vi "Read File.vi"(8 "error in (no error)":errorcluster, 11 "Context in":T1 {"Progress" scale=0.0..100.0}) -> (0 "error out":errorcluster, 3 "Context out":T1 {"Progress" scale=0.0..100.0})   [LabVIEW 2020, in "DocTool.lvlib"]
uses:
  DocTool.lvlib
  TDefs/Context.ctl
  Events.ctl
  UserEvent.ctl
  TDefs/State.ctl
  TDefs/States.ctl
  TDefs/Single File Properties.ctl
  TDefs/FP Items Properties.ctl
  TDefs/FP Item Properties.ctl
  TDefs/CopyTag.ctl
  StateMachine.lvlib
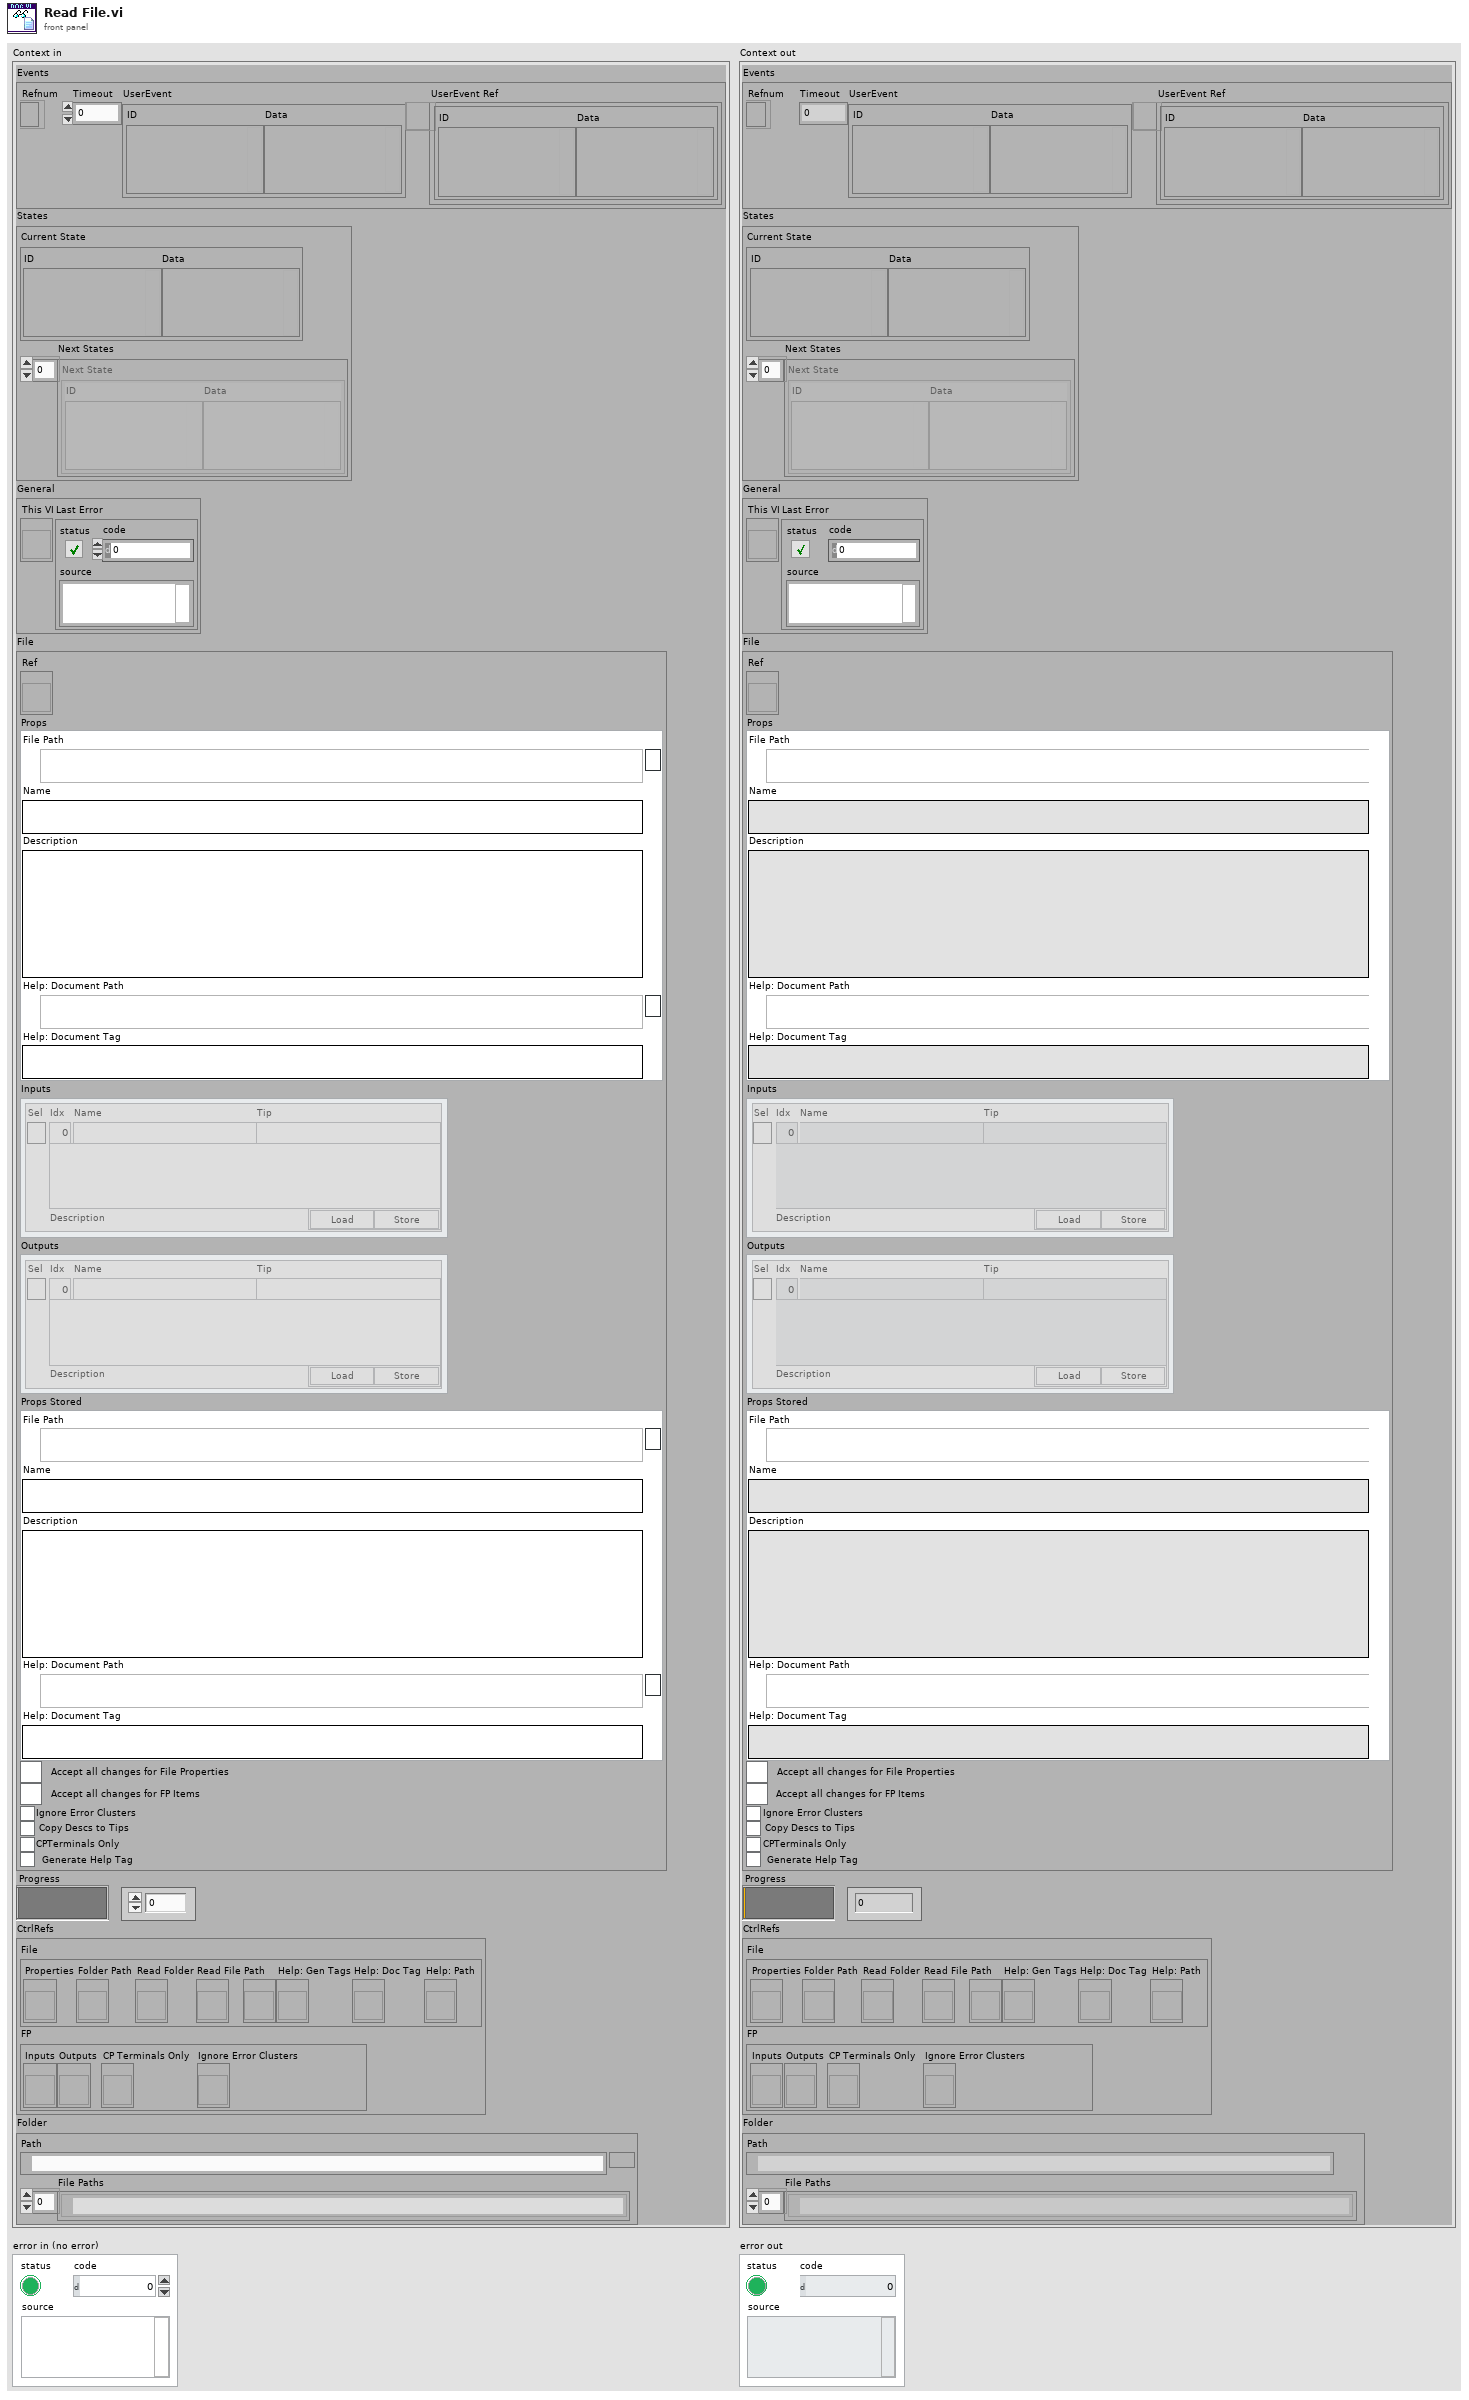
[diagram p1: front panel]
types:
  T1 = typedef "DocTool.lvlib/Context.ctl" = cluster{"Events":T2, "States":cluster{"Current State":T4, "Next States":T5}, "General":cluster{"This VI":refnum<vi>, "Last Error":errorcluster}, "File":cluster{"Ref":refnum<vi>, "Props":T6, "Inputs":T7, "Outputs":T7, "Props Stored":T6, "Write":bool, "Write FP":bool, "Ignore Error Clusters":bool, "Copy Descs to Tips":bool, "CPTerminals Only":bool, "Generate Help Tag":bool}, "Progress":i32, "CtrlRefs":cluster{"File":cluster{"Properties":refnum<vi>, "Folder Path":refnum<vi>, "Read Folder":refnum<vi>, "Read File":refnum<vi>, "Path":refnum<vi>, "Help: Gen Tags":refnum<vi>, "Help: Doc Tag":refnum<vi>, "Help: Path":refnum<vi>}, "FP":cluster{"Inputs":refnum<vi>, "Outputs":refnum<vi>, "CP Terminals Only":refnum<vi>, "Ignore Error Clusters":refnum<vi>}}, "Folder":cluster{"Path":path, "File Paths":path[]}}
  T2 = typedef "StateMachine.lvlib/Events.ctl" = cluster{"Refnum":refnum<event-registration>, "Timeout":i32, "UserEvent":T3, "UserEvent Ref":refnum<user-event>}
  T3 = typedef "StateMachine.lvlib/UserEvent.ctl" = cluster{"ID":variant, "Data":variant}
  T4 = typedef "StateMachine.lvlib/State.ctl" = cluster{"ID":variant, "Data":variant}
  T5 = typedef "StateMachine.lvlib/States.ctl" = T4[]
  T6 = typedef "DocTool.lvlib/Single File Properties.ctl" = cluster{"File Path":path, "Name":string, "Description":string, "Help: Document Path":path, "Help: Document Tag":string}
  T7 = typedef "DocTool.lvlib/FP Items Properties.ctl" = T8[]
  T8 = typedef "DocTool.lvlib/FP Item Properties.ctl" = cluster{"Sel":bool, "Idx":i32, "Name":string, "Description":string, "Tip":string, "Load Store":T9}
  T9 = typedef "DocTool.lvlib/CopyTag.ctl" = cluster{"Load":bool, "Store":bool}
  T10 = enum8{"Enabled", "Disabled", "Disabled and Grayed Out"}
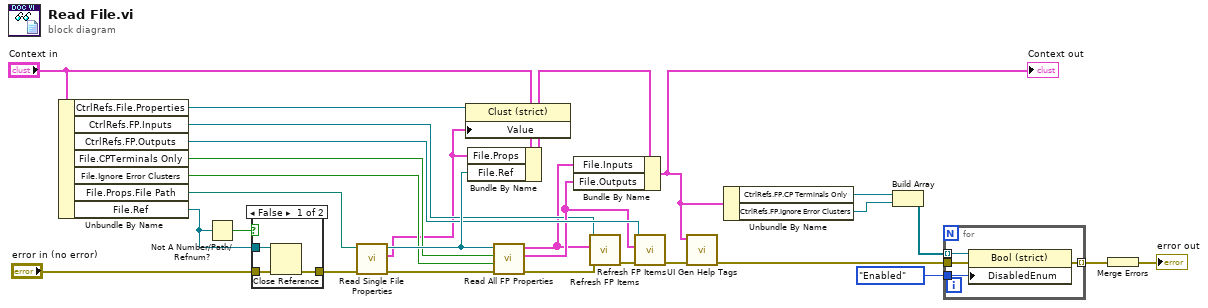
[diagram p0: block diagram]
diagram:
  n1 = Unbundle By Name("Context in") -> ("CtrlRefs.File.Properties"=w17:refnum<vi>, "CtrlRefs.FP.Inputs"=w20:refnum<vi>, "CtrlRefs.FP.Outputs"=w23:refnum<vi>, "File.CPTerminals Only"=w24:bool, "File.Ignore Error Clusters"=w26:bool, "File.Props.File Path"=w13:path, "File.Ref"=w10:refnum<vi>)
  n2 = Not A Number/Path/Refnum?(number/path/refnum=w10) -> (NaN/Path/Refnum?=w9:bool)
  n3 = case shown="False" w9 {
    tunnel: w10 -> [w31 _]
    tunnel: "error in (no error)" -> [w30 w32]
    tunnel: [w29 w32] -> w11
    frame False {
      n4 = Close Reference(reference=w31, error in (no error)=w30) -> (error out=w29:errorcluster)
    }
    frame True {
    }
  }
  n5 = call "Read Single File Properties.vi"("error in (no error)"=w11, "File Path"=w13) -> ("error out"=w15:errorcluster, "File Properties"=w18:T6, "File Ref"=w27:refnum<vi>)  [unwired: 7 in]
  n6 = property class="Clust (strict)"(reference=w17, "Value"=w18) -> ()  [unwired: 1 in, 2 out]
  n7 = Bundle By Name(cluster="Context in", "File.Props"=w18, "File.Ref"=w27) -> (w16:T1)
  n8 = call "Read All FP Properties.vi"("error in (no error)"=w15, "No Error clusters"=w26, "Is On Connector Pane"=w24, "VI in"=w27) -> ("error out"=w25:errorcluster, "Outputs"=w22:T7, "Inputs"=w19:T7)  [unwired: 5 in]
  n9 = Bundle By Name(cluster=w16, "File.Inputs"=w19, "File.Outputs"=w22) -> (w5:T1)
  "Context out" <- w5
  n10 = call "Refresh FP Items.vi"("error in (no error)"=w25, "FP Item Props in"=w19, "Array in"=w20) -> ("error out"=w21:errorcluster)  [unwired: 8 in]
  n11 = call "Refresh FP Items.vi"("error in (no error)"=w21, "FP Item Props in"=w22, "Array in"=w23) -> ("error out"=w28:errorcluster)  [unwired: 8 in]
  n12 = call "UI Gen Help Tags.vi"("error in (no error)"=w28, "Context"=w5) -> ("error out"=w4:errorcluster)  [unwired: 9 in]
  n13 = Unbundle By Name(w5) -> ("CtrlRefs.FP.CP Terminals Only"=w7:refnum<vi>, "CtrlRefs.FP.Ignore Error Clusters"=w3:refnum<vi>)
  n14 = Build Array(w7, w3) -> (w6:refnum<vi>[])
  n15 = for {
    tunnel: w6 -> [w36] mode=indexing
    tunnel: w4 -> [w35]
    tunnel: [w34] -> w2 mode=indexing
    tunnel: T10."Enabled" ("Disabled") -> [w33]
    n16 = property class="Bool (strict)"(reference=w36, error in=w35, "DisabledEnum"=w33) -> (error out=w34:errorcluster)  [unwired: 1 out]
  }
  n17 = Merge Errors(w2) -> (→"error out":errorcluster)
